vi "LV type to MCP type.vi"(11 "type":T1) -> (2 "Valid?":bool, 3 "JSON to Insert":string)   [LabVIEW 2025, in "MCP Server.lvlib"]
uses:
  MCP Server.lvlib
  <vilib>/Utility/Data Type/Type Definitions/Data Type.ctl
  <vilib>/Utility/Data Type/NI_Data Type.lvlib
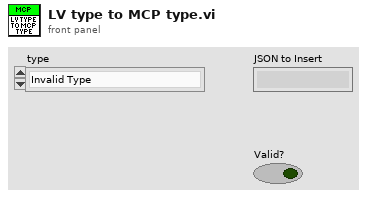
[diagram p1: front panel]
types:
  T1 = typedef "NI_Data Type.lvlib/Data Type.ctl" = enum8{"Invalid Type", "Void", "I8", "I16", "I32", "I64", "U8", "U16", "U32", "U64", "Single Float", "Double Float", "Extended Float", "Single Complex", "Double Complex", "Extended Complex", "Enum U8", "Enum U16", "Enum U32", "Enum U64", "Single Float With Unit", "Double Float With Unit", "Extended Float With Unit", "Single Complex with Unit", "Double Complex with Unit", "Extended Complex with Unit", "Boolean", "String", "Path", "Picture", "Tag", "Array", "Cluster", "Variant", "LV Variant", "Waveform", "Timestamp", "Digital Waveform", "Digital Data", "ExpressData", "Refnum", "External Data", "VI", "Poly VI", "LabVIEW Class Instance", "Fixed Point", "Set Collection", "Map Collection"}
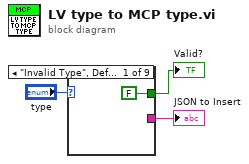
[diagram p0: block diagram]
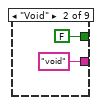
[diagram p2: hidden frame]
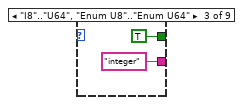
[diagram p3: hidden frame]
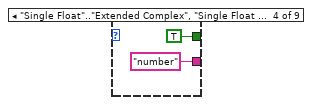
[diagram p4: hidden frame]
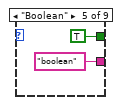
[diagram p5: hidden frame]
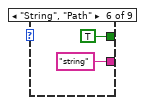
[diagram p6: hidden frame]
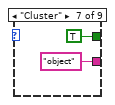
[diagram p7: hidden frame]
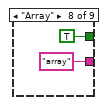
[diagram p8: hidden frame]
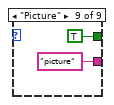
[diagram p9: hidden frame]
diagram:
  n1 = case shown="\"Invalid Type\", Default" "type" {
    tunnel: [_ "void" ("JSON to Insert") "integer" ("JSON to Insert") "number" ("JSON to Insert") "boolean" ("JSON to Insert") "string" ("JSON to Insert") "object" ("JSON to Insert") "array" ("JSON to Insert") "picture" ("JSON to Insert")] -> w3
    tunnel: [FALSE FALSE TRUE TRUE TRUE TRUE TRUE TRUE TRUE] -> w2
    frame "Invalid Type", Default {
    }
    frame "Void" {
    }
    frame "I8".."U64", "Enum U8".."Enum U64" {
    }
    frame "Single Float".."Extended Complex", "Single Float With Unit".."Extended Complex with Unit" {
    }
    frame "Boolean" {
    }
    frame "String", "Path" {
    }
    frame "Cluster" {
    }
    frame "Array" {
    }
    frame "Picture" {
    }
  }
  "JSON to Insert" <- w3
  "Valid?" <- w2
